vi "userOperationDisplay.vi"(8 "error in (no error)":errorcluster, 10 "Current User Operation":string, 11 "Management in":refnum<class "Display.lvclass">) -> (0 "error out":errorcluster, 3 "Management out":refnum<class "Display.lvclass">)   [LabVIEW 2015, in "UserManagement.lvlib" / "Display.lvclass"]
doc: "Functions: <b> In this VI, we send all msg about user operation in our front panel!"
uses:
  Display.lvclass
  Display.lvclass/Display.ctl
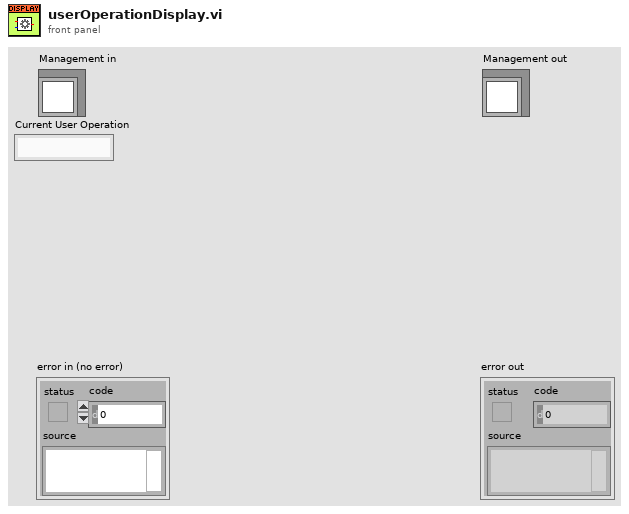
[diagram p1: front panel]
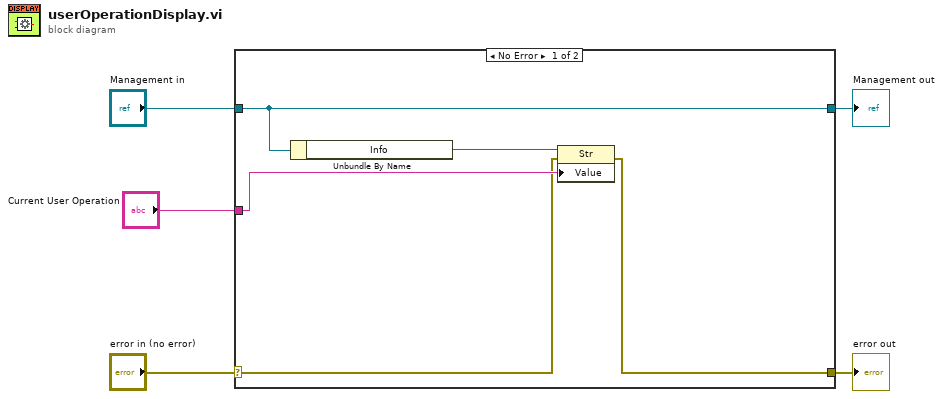
[diagram p0: block diagram]
diagram:
  n1 = case shown="No Error" "error in (no error)" {
    selector: "error in (no error)" -> [w7 w12]
    tunnel: [w6 w12] -> w4
    tunnel: [w10 w11] -> w2
    tunnel: "Management in" -> [w10 w11]
    tunnel: "Current User Operation" -> [w8 _]
    frame No Error {
      n2 = Unbundle By Name(w10) -> ("Info"=w9:refnum<vi>)
      n3 = property class="Str"(reference=w9, error in=w7, "Value"=w8) -> (error out=w6:errorcluster)  [unwired: 1 out]
    }
    frame Error {
    }
  }
  "error out" <- w4
  "Management out" <- w2
